vi "Begin.vi"(8 "error in (no error)":errorcluster, 11 "EventMgr in":refnum<class "EventMgr.lvclass">) -> (0 "error out":errorcluster, 3 "EventMgr out":refnum<class "EventMgr.lvclass">)   [LabVIEW 2013, in "EventMgr.lvclass"]
uses:
  EventMgr.lvclass
  Utilities/Event/Event.lvclass
  EventMgr.lvclass/EventMgr.ctl
  System/System.lvclass
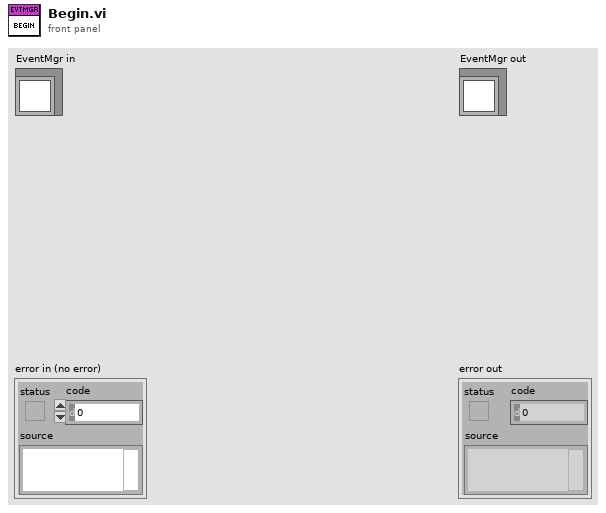
[diagram p1: front panel]
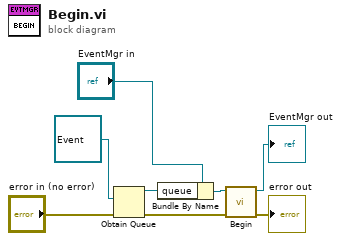
[diagram p0: block diagram]
diagram:
  n1 = Obtain Queue(element data type=refnum<class "Event.lvclass"> refnum ("Event.lvclass"), error in (no error)="error in (no error)") -> (queue out=w1:refnum<queue>, error out=w3:errorcluster)  [unwired: 3 in, 1 out]
  n2 = Bundle By Name(cluster="EventMgr in", "queue"=w1) -> (w2:refnum<class "EventMgr.lvclass">)
  n3 = call-parent "Begin.vi"("error in (no error)"=w3, "System in"=w2) -> ("error out"=→"error out":errorcluster, "System out"=→"EventMgr out":refnum<class "EventMgr.lvclass">)  [unwired: 8 in]
